vi "Frame to Send.vi"(8 "error in (no error)":errorcluster caption="entrée d'erreur (pas d'erreur)", 10 "Number Prog":string, 11 "Class Camera  IV3-500CA - Start Program en Entrée":refnum<class "Class Camera  Commande (Default).lvclass">) -> (0 "error out":errorcluster caption="sortie d'erreur", 2 "Frame to Write":string, 3 "Class Camera  IV3-500CA - Start Program en Sortie":refnum<class "Class Camera  Commande (Default).lvclass">)   [LabVIEW 2020, in "Library Instrument & Equipement.lvlib" / "Library Camera.lvlib" / "Class Camera  Commande (Default).lvclass"]
uses:
  Class Camera  Commande (Default).lvclass
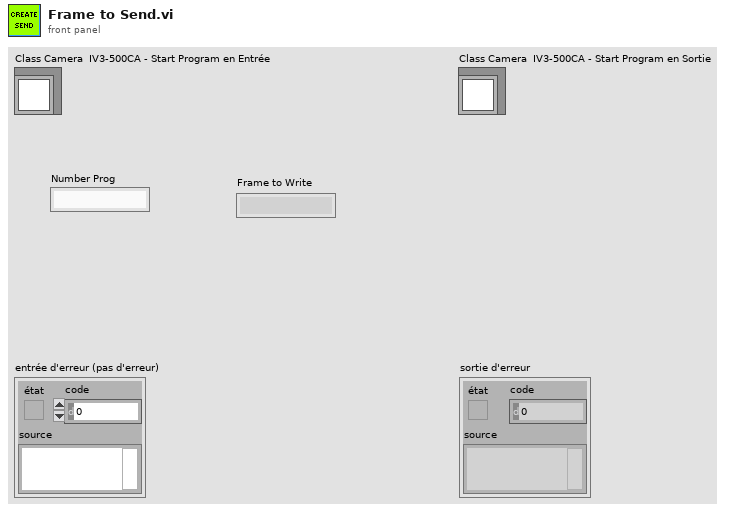
[diagram p1: front panel]
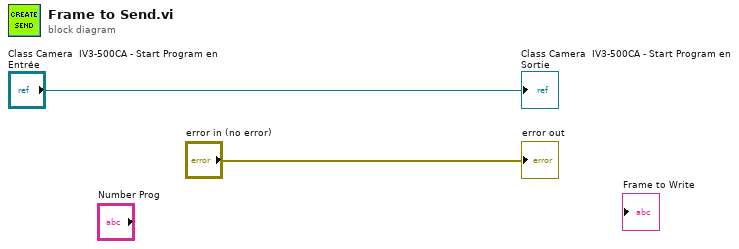
[diagram p0: block diagram]
diagram:
  "error out" <- "error in (no error)"
  "Class Camera  IV3-500CA - Start Program en Sortie" <- "Class Camera  IV3-500CA - Start Program en Entrée"
